vi "MyG#SubClass_Create.vi"(0 "reference in":refnum<class "MyG#SubClass.lvclass">, 1 "MySubAttribute":dbl, 2 "MyAttribute":dbl, 5 "error in (no error)":errorcluster, 6 "object name":string, 7 "user counter":bool=TRUE) -> (14 "reference out":refnum<class "MyG#SubClass.lvclass">, 19 "error out":errorcluster)   [LabVIEW 2020, in "MyG#SubClass.lvclass"]
doc: "Constructor."
uses:
  MyG#SubClass.lvclass
  C:/Program Files (x86)/National Instruments/LabVIEW 2020/vi.lib/addons/_AddQ/G#Object/G#Object.lvclass
  C:/Program Files (x86)/National Instruments/LabVIEW 2020/examples/AddQ/G#/CreateDestroy/MyG#Class_class/MyG#Class.lvclass
  vi.lib/addons/_AddQ/G#Object/utils/G#Object_CreateMethod.ctl
  vi.lib/addons/_AddQ/G#Object/G#Object.lvclass
  MyG#Class_class/MyG#Class.lvclass
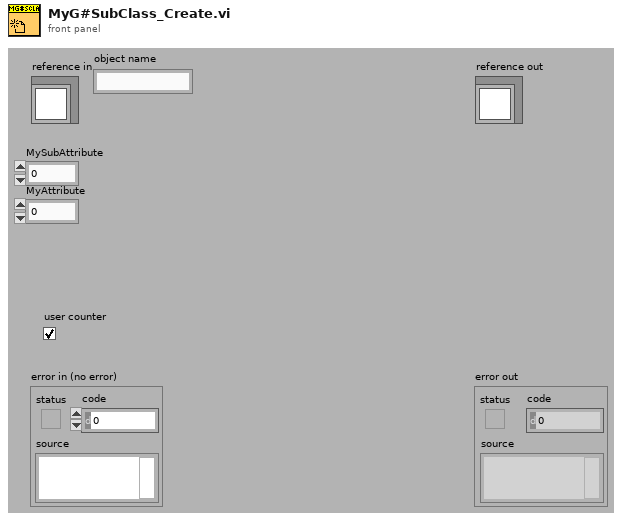
[diagram p1: front panel]
types:
  T1 = typedef "G#Object.lvclass/G#Object_CreateMethod.ctl" = enum16{"Create", "Create or look up existing", "Look up existing"}
  T2 = typedef "MyG#SubClass.lvclass/ObjectAttributesRef.ctl" = refnum<data-value>
  T3 = typedef "MyG#SubClass.lvclass/ObjectAttributes.ctl" = cluster{"MySubAttribute":dbl}
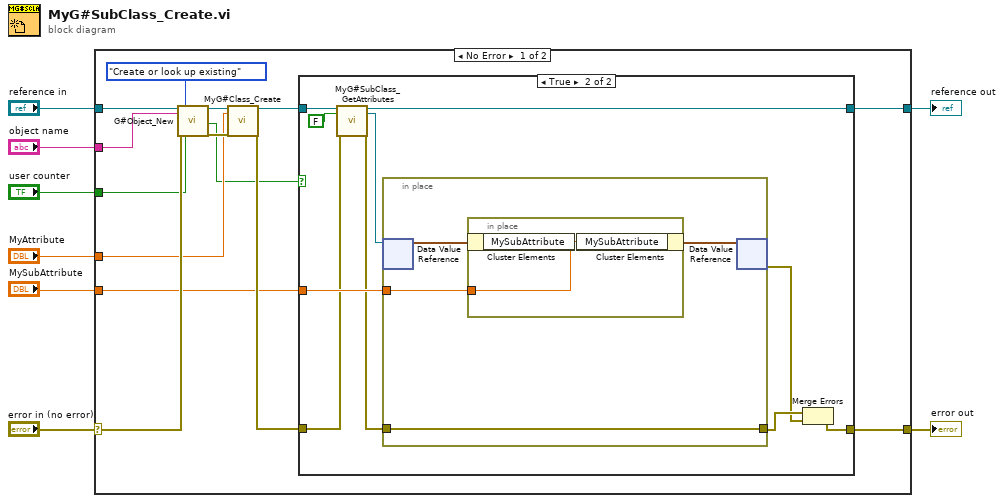
[diagram p0: block diagram]
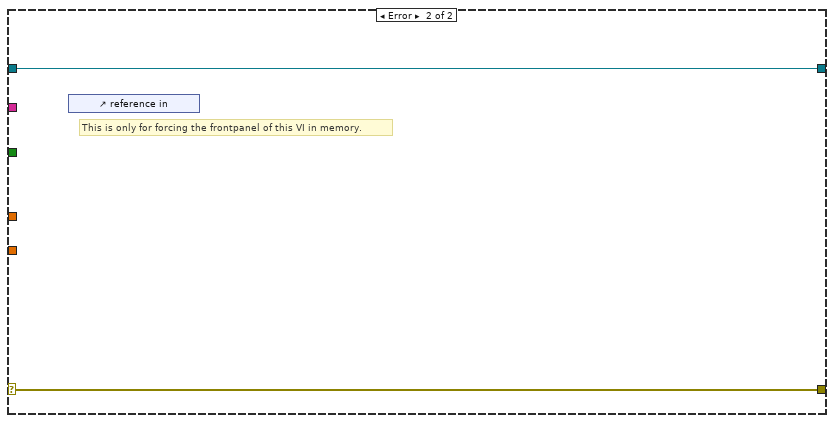
[diagram p3: hidden frame]
diagram:
  n1 = case shown="No Error" "error in (no error)" {
    selector: "error in (no error)" -> [w21 w41]
    tunnel: [w20 w41] -> w7
    tunnel: [w9 w40] -> w5
    tunnel: "reference in" -> [w22 w40]
    tunnel: "MySubAttribute" -> [w16 _]
    tunnel: "MyAttribute" -> [w15 _]
    tunnel: "object name" -> [w13 _]
    tunnel: "user counter" -> [w12 _]
    frame No Error {
      n2 = call "G#Object_New.vi"("reference in"=w22, "object name"=w13, "error in (no error)"=w21, "create method"=G#Object_CreateMethod."Create or look up existing", "user counter (T)?"=w12) -> ("reference out"=w19:refnum<class "MyG#SubClass.lvclass">, "created new?"=w11:bool, "error out"=w18:errorcluster)  [unwired: 12 in]
      n3 = call "MyG#Class_Create.vi"("reference in"=w19, "MyAttribute"=w15, "error in (no error)"=w18) -> ("reference out"=w10:refnum<class "MyG#SubClass.lvclass">, "error out"=w17:errorcluster)  [unwired: 15 in]
      n4 = case shown="True" w11 {
        tunnel: [w24 w34] -> w20
        tunnel: w17 -> [w24 w29]
        tunnel: w16 -> [_ w31]
        tunnel: w10 -> [w23 w30]
        tunnel: [w23 w26] -> w9
        frame False {
          # "I am not the first user of this object! Don't initialize the attributes!"
        }
        frame True {
          n5 = call "MyG#SubClass_GetAttributes.vi"("reference in"=w30, "return data? (T)"=FALSE, "error in (no error)"=w29) -> ("reference out"=w26:refnum<class "MyG#SubClass.lvclass">, "attributes ref"=w25:T2, "error out"=w28:errorcluster)  [unwired: 13 in, 1 out]
          n6 = in-place {
            in-place-border: w28 -> [w36]
            in-place-border: [w36] -> w33
            in-place-border: w31 -> [w35]
            n7 = in-place-dvr #1(w25) -> (w37:T3)  [unwired: 1 out]
            n8 = in-place {
              in-place-border: w35 -> [w39]
              n9 = in-place-cluster #2(w37) -> ()  [unwired: 1 out]
              n10 = in-place-cluster #2("MySubAttribute"=w39) -> (w38:T3)
            }
            n11 = in-place-dvr #1(w38) -> (w32:errorcluster)  [unwired: 1 out]
          }
          n12 = Merge Errors(w33, w32) -> (w34:errorcluster)
        }
      }
    }
    frame Error {
      # "This is only for forcing the frontpanel of this VI in memory."
      n13 = control-ref of="reference in"() -> ()  [unwired: 1 out]
    }
  }
  "error out" <- w7
  "reference out" <- w5
